vi "OPO_TCP_Server.vi"(0 "address":string="localhost", 1 "port":u16=6000, 2 "OPO Value":dbl=261.0, 3 "error in (no error)":errorcluster) -> (10 "error out":errorcluster)   [LabVIEW 2024]
panel:
  out "length":i32
  out "data read":string
  out "bytes written":i32
  out "byte written length":i32
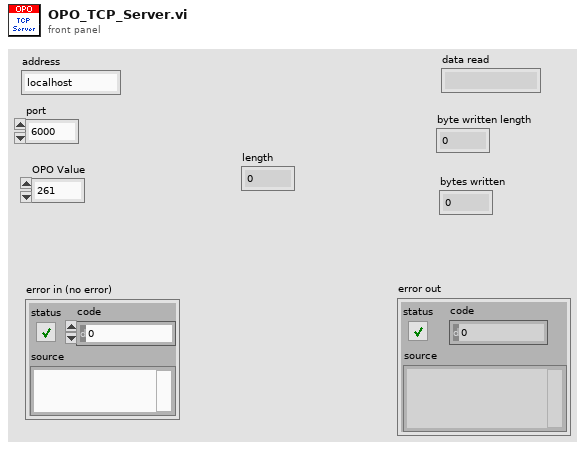
[diagram p1: front panel]
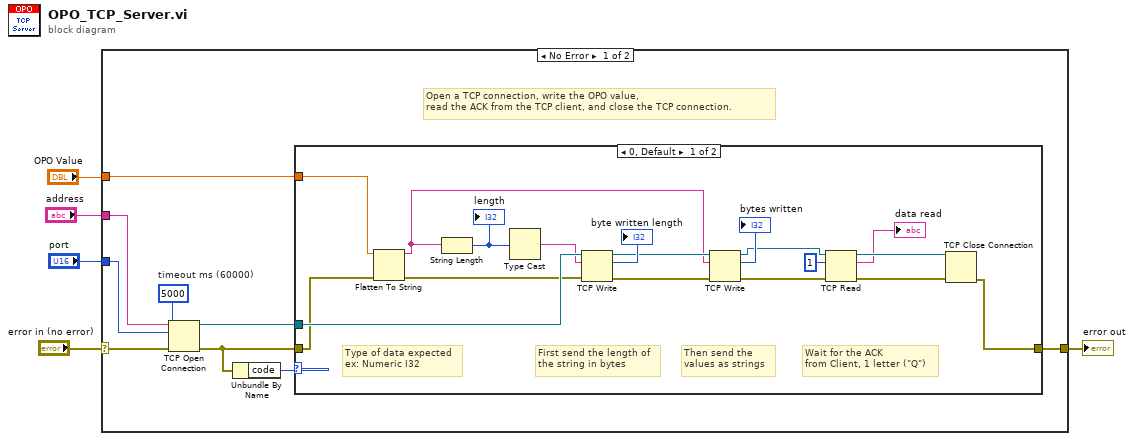
[diagram p0: block diagram]
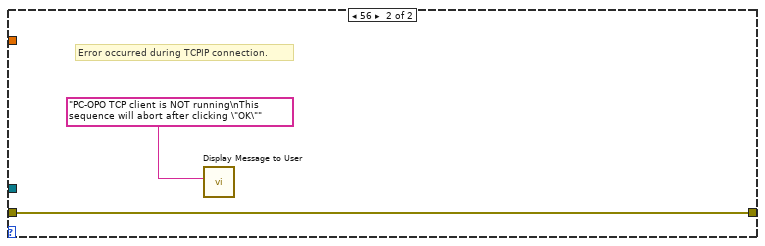
[diagram p2: hidden frame]
diagram:
  n1 = case shown="No Error" "error in (no error)" {
    selector: "error in (no error)" -> [w13 w35]
    tunnel: [w12 w35] -> w4
    tunnel: "port" -> [w14 _]
    tunnel: "address" -> [w11 _]
    tunnel: "OPO Value" -> [w10 _]
    frame No Error {
      w8 = 5000  # timeout ms (60000)
      # "Open a TCP connection, write the OPO value,\nread the ACK from the TCP client, and close the TCP connection."
      n2 = TCP Open Connection(address=w11, remote port or service name=w14, timeout ms (60000)=w8, error in (no error)=w13) -> (connection ID=w9:refnum<k5>, error out=w6:errorcluster)  [unwired: 1 in]
      n3 = Unbundle By Name(w6) -> ("code"=w7:i32)
      n4 = case shown="0, Default" w7 {
        tunnel: [w32 w33] -> w12
        tunnel: w10 -> [w31 _]
        tunnel: w9 -> [w30 _]
        tunnel: w6 -> [w15 w33]
        frame 0, Default {
          # "Wait for the ACK\nfrom Client, 1 letter (\"Q\")"
          # "Then send the values as strings"
          # "First send the length of\nthe string in bytes"
          # "Type of data expected\nex: Numeric I32"
          n5 = Flatten To String(anything=w31, error in (no error)=w15) -> (data string=w20:string, error out=w27:errorcluster)  [unwired: 2 in, 1 out]
          n6 = String Length(string=w20) -> (length=w25:i32)
          "length" <- w25
          n7 = Type Cast(x=w25) -> (*(type *) &x=w24:string)  [unwired: 1 in]
          n8 = TCP Write(connection ID=w30, data in=w24, error in (no error)=w27) -> (connection ID out=w21:refnum<k5>, bytes written=→"byte written length":i32, error out=w26:errorcluster)  [unwired: 1 in]
          n9 = TCP Write(connection ID=w21, data in=w20, error in (no error)=w26) -> (connection ID out=w16:refnum<k5>, bytes written=→"bytes written":i32, error out=w22:errorcluster)  [unwired: 1 in]
          n10 = TCP Read(connection ID=w16, bytes to read=1, error in (no error)=w22) -> (connection ID out=w28:refnum<k5>, data out=→"data read":string, error out=w29:errorcluster)  [unwired: 2 in]
          n11 = TCP Close Connection(connection ID=w28, error in (no error)=w29) -> (error out=w32:errorcluster)  [unwired: 1 in, 1 out]
        }
        frame 56 {
          # "Error occurred during TCPIP connection."
          n12 = call "Display Message to User"("Message"="PC-OPO TCP client is NOT running\nThis sequence will abort after clicking \"OK\"") -> ()  [unwired: 9 in, 2 out]
        }
      }
    }
    frame Error {
    }
  }
  "error out" <- w4
